vi "Generator_cosinusa.vi"(10 "Parametry_cosinusa":T1, 11 "Czas":dbl) -> (3 "A cos(2pift + phi)":dbl)   [LabVIEW 2020]
doc: "VI zwraca wartosci sygnalu cosinusoidalnego"
uses:
  Kontrolki/Parametry_cosinusa.ctl
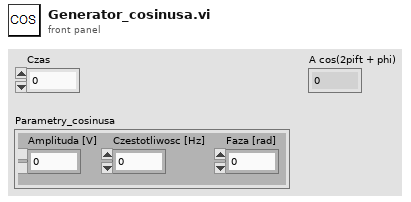
[diagram p1: front panel]
types:
  T1 = typedef "Parametry_cosinusa.ctl" = cluster{"Amplituda [V]":dbl, "Czestotliwosc [Hz] ":dbl, "Faza [rad]":dbl}
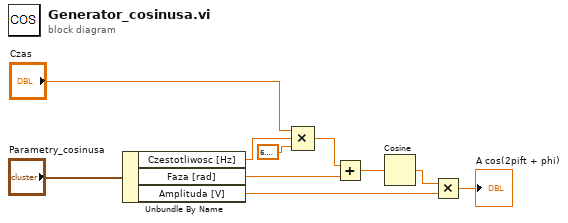
[diagram p0: block diagram]
diagram:
  n1 = Unbundle By Name("Parametry_cosinusa") -> ("Czestotliwosc [Hz]"=w3:dbl, "Faza [rad]"=w6:dbl, "Amplituda [V]"=w9:dbl)
  n2 = Compound Arithmetic op=MULTIPLY("Czas", w3, 6.283185307179586) -> (w5:dbl)
  n3 = Add(x=w5, y=w6) -> (x+y=w7:dbl)
  n4 = Cosine(x=w7) -> (cos(x)=w8:dbl)
  n5 = Multiply(x=w8, y=w9) -> (x*y=→"A cos(2pift + phi)":dbl)
